vi "robot_state.vi"(11 "Topic Name":string="rt/robot_state") -> (3 "Int from ros":i32)   [LabVIEW 2024]
uses:
  <vilib>/RTI DDS Toolkit/Types/RTI DDS Advanced Reader Configuration.ctl
  <vilib>/RTI DDS Toolkit/VIs/AdvancedCreateReader_NumI32.vi
  <vilib>/RTI DDS Toolkit/VIs/Read_NumI32.vi
  <vilib>/RTI DDS Toolkit/Library/LVDDS_library.lvlib
panel:
  in  "Data Type":i32
  in  "Domain id":u32
  in  "stop":bool
  in  "error in (no error)":errorcluster
  in  "Advanced Reader Configuration":T1={"typeName"="std_msgs::msg::dds_::Int32_", "keyName"="", "domainParticipantQoSProfile"="", "dataReaderQoSProfile"="", "forceArrayMapping?"=FALSE, "forceExclusiveReader?"=FALSE, "forceRead? (only ExclusiveReader)"=FALSE, "forceUnboundedString?"=FALSE}
  # "Robot state from ROS Topic over DDS"
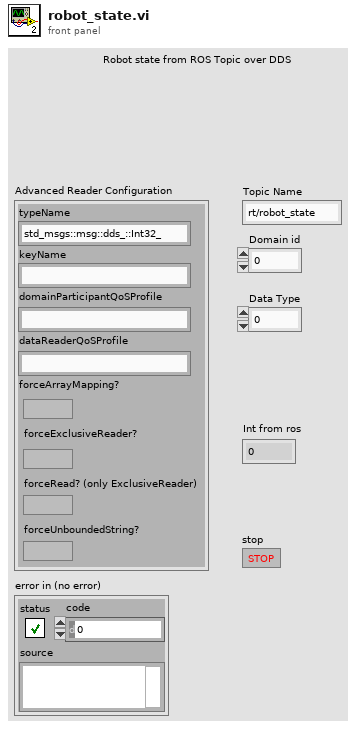
[diagram p1: front panel]
types:
  T1 = typedef "LVDDS_library.lvlib/RTI DDS Advanced Reader Configuration.ctl" = cluster{"typeName":string, "keyName":string, "domainParticipantQoSProfile":string, "dataReaderQoSProfile":string, "forceArrayMapping?":bool, "forceExclusiveReader?":bool, "forceRead? (only ExclusiveReader)":bool, "forceUnboundedString?":bool}
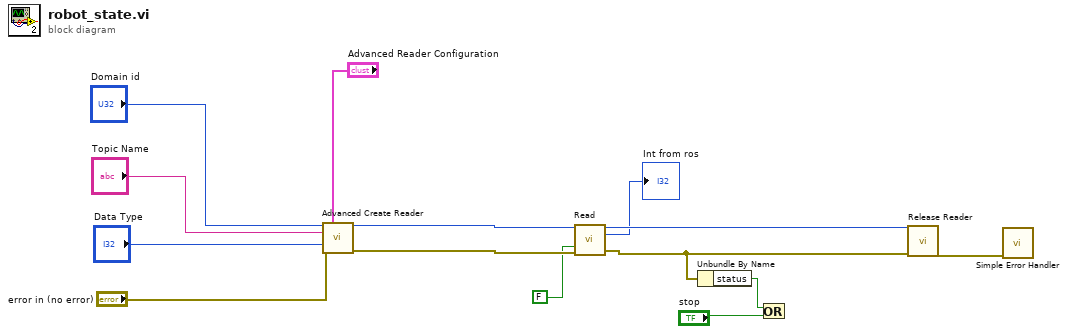
[diagram p0: block diagram]
diagram:
  n1 = call-poly <vilib>:"Advanced Create Reader.vi"("Domain Id"="Domain id", "Advanced Reader Configuration"="Advanced Reader Configuration", "Topic Name"="Topic Name", "Data Type"="Data Type", "error in (no error)"="error in (no error)") -> ("DDS Object Ref"=w9:u64, "error out"=w8:errorcluster)  [unwired: 9 in]
  n2 = call-poly <vilib>:"Read.vi"("DDS Object Ref in"=w9, "Only New Samples"=FALSE, "error in (no error)"=w8) -> ("DDS Object Ref out"=w7:u64, "Data"=→"Int from ros":i32, "error out"=w6:errorcluster)  [unwired: 8 in, 2 out]
  n3 = Unbundle By Name(w6) -> ("status"=w2:bool)
  n4 = Or(x=w2, y="stop") -> ()  [unwired: 1 out]
  n5 = call <vilib>:"Release Reader.vi"("error in (no error)"=w6, "DDS Object Ref"=w7) -> ("error out"=w5:errorcluster)  [unwired: 9 in]
  n6 = call <vilib>:"Simple Error Handler.vi"("error in (no error)"=w5) -> ()  [unwired: 4 in, 5 out]
